vi "Ctor.vi"(8 "error in (no error)":errorcluster, 11 "ByRef Add in":refnum<class "ByRef Add.lvclass">) -> (0 "error out":errorcluster, 3 "ByRef Add out":refnum<class "ByRef Add.lvclass">)   [LabVIEW 2020, in "ByRef Add.lvclass"]
uses:
  ByRef Add.lvclass
  Ref Data.ctl
  ByRef Add.lvclass/ByRef Add.ctl
  ByRef Base/ByRef Base.lvclass
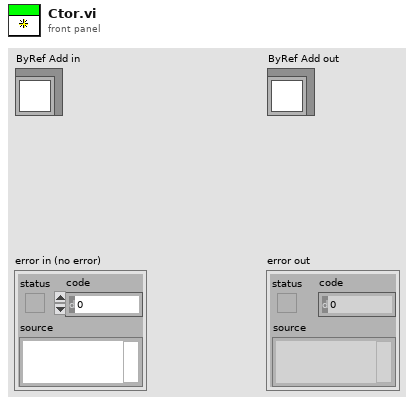
[diagram p1: front panel]
types:
  T1 = typedef "ByRef Add.lvclass/Ref Data.ctl" = cluster{"String":string}
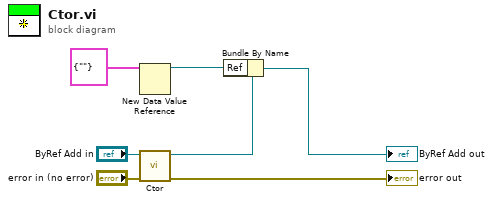
[diagram p0: block diagram]
diagram:
  n1 = New Data Value Reference(data value=T1 {"String"=""} ("Ref Data")) -> (data value reference=w1:refnum<data-value>)  [unwired: 1 in, 1 out]
  n2 = call-parent "Ctor.vi"("error in (no error)"="error in (no error)", "ByRef Base in"="ByRef Add in") -> ("error out"=→"error out":errorcluster, "ByRef Base out"=w6:refnum<class "ByRef Add.lvclass">)  [unwired: 8 in]
  n3 = Bundle By Name(cluster=w6, "Ref"=w1) -> (→"ByRef Add out":refnum<class "ByRef Add.lvclass">)
